vi "motorJoystickcore.vi"(4 "button info":T2, 6 "axis info":T1, 8 "error in":errorcluster[](array[cluster]), 9 "Motor Limits":T3, 10 "Array in":refnum<k7>[](array[refnum])) -> (0 "error out":errorcluster[](array[cluster]), 2 "XYZ position":sgl[](array[numeric]))   [LabVIEW 2014]
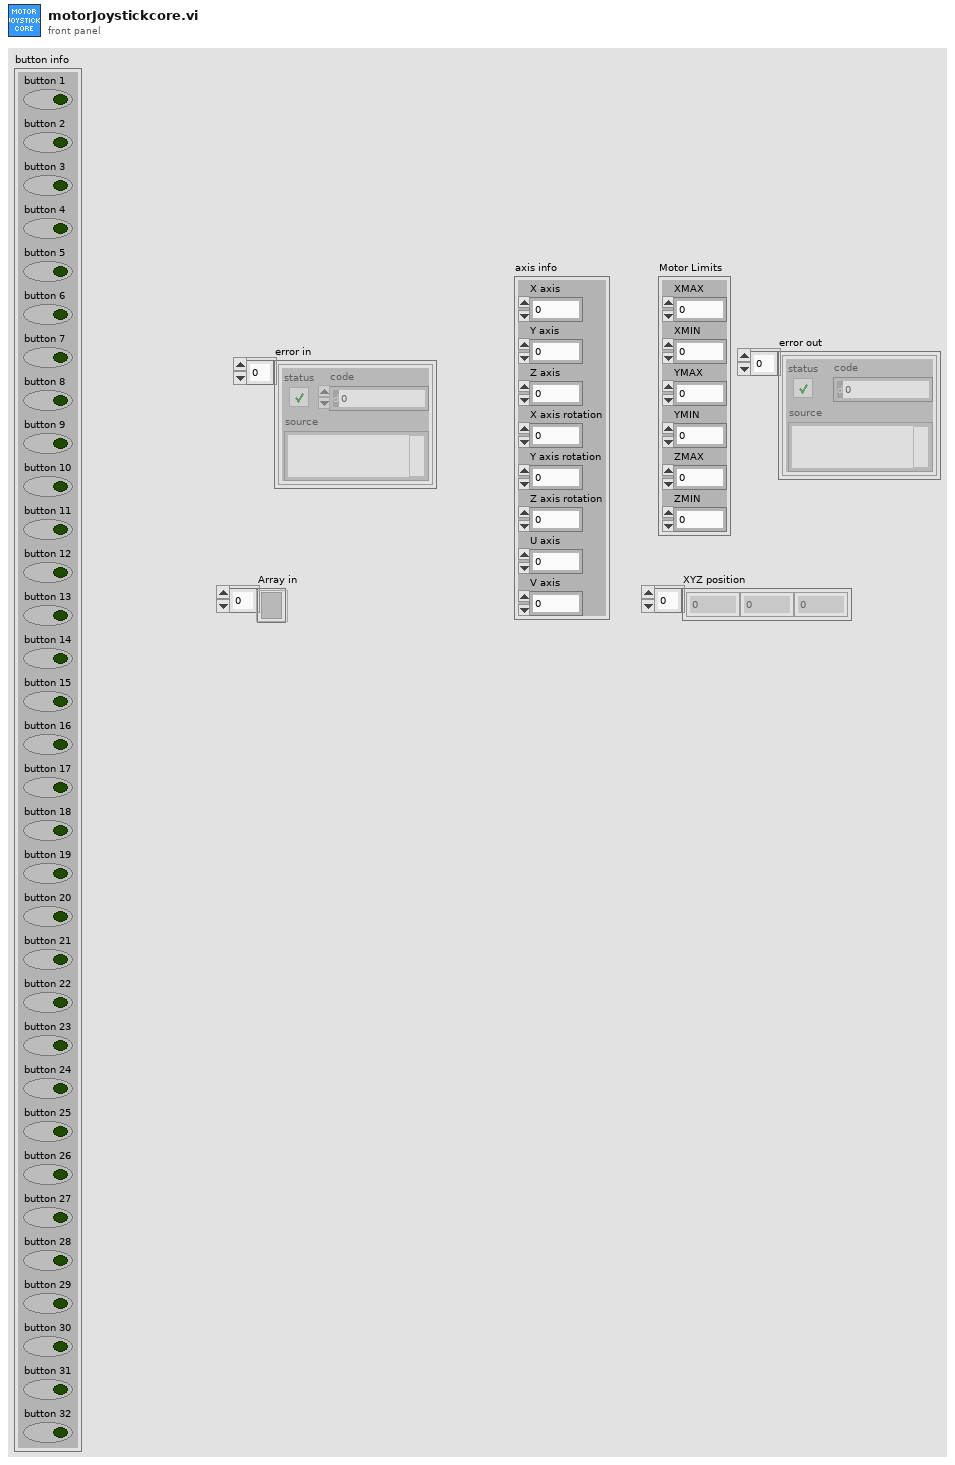
[diagram p1: front panel]
types:
  T1 = cluster{"X axis":i32, "Y axis":i32, "Z axis":i32, "X axis rotation":i32, "Y axis rotation":i32, "Z axis rotation":i32, "U axis":i32, "V axis":i32}
  T2 = cluster{"button 1":bool, "button 2":bool, "button 3":bool, "button 4":bool, "button 5":bool, "button 6":bool, "button 7":bool, "button 8":bool, "button 9":bool, "button 10":bool, "button 11":bool, "button 12":bool, "button 13":bool, "button 14":bool, "button 15":bool, "button 16":bool, "button 17":bool, "button 18":bool, "button 19":bool, "button 20":bool, "button 21":bool, "button 22":bool, "button 23":bool, "button 24":bool, "button 25":bool, "button 26":bool, "button 27":bool, "button 28":bool, "button 29":bool, "button 30":bool, "button 31":bool, "button 32":bool}
  T3 = cluster{"XMAX":sgl, "XMIN":sgl, "YMAX":sgl, "YMIN":sgl, "ZMAX":sgl, "ZMIN":sgl}
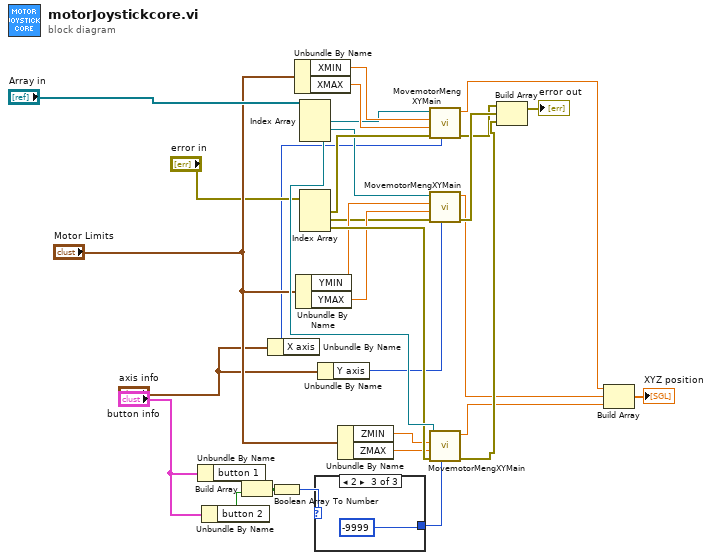
[diagram p0: block diagram]
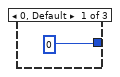
[diagram p2: hidden frame]
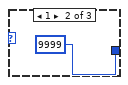
[diagram p3: hidden frame]
diagram:
  n1 = Unbundle By Name("button info") -> ("button 1"=w8:bool)
  n2 = Unbundle By Name("button info") -> ("button 2"=w9:bool)
  n3 = Build Array(w8, w9) -> (w10:bool[])
  n4 = Unbundle By Name("axis info") -> ("X axis"=w6:i32)
  n5 = Boolean Array To Number(Boolean array=w10) -> (number=w11:u32)
  n6 = Unbundle By Name("Motor Limits") -> ("XMIN"=w21:sgl, "XMAX"=w22:sgl)
  n7 = Unbundle By Name("Motor Limits") -> ("YMIN"=w23:sgl, "YMAX"=w24:sgl)
  n8 = Index Array(array="Array in") -> (element #1=w13:refnum<k7>, element #2=w14:refnum<k7>, element #3=w32:refnum<k7>)  [unwired: 3 in]
  n9 = Index Array(array="error in") -> (element #1=w16:errorcluster, element #2=w17:errorcluster, element #3=w29:errorcluster)  [unwired: 3 in]
  n10 = case shown="2" w11 {
    tunnel: [0 ("Y axis") 9999 ("Y axis") -9999 ("Y axis")] -> w12
    frame 0, Default {
    }
    frame 1 {
    }
    frame 2 {
    }
  }
  n11 = Unbundle By Name("axis info") -> ("Y axis"=w7:i32)
  n12 = Unbundle By Name("Motor Limits") -> ("ZMIN"=w25:sgl, "ZMAX"=w26:sgl)
  n13 = call "MovemotorMengXYMain.vi"("Joystick axis"=w6, "error in (no error)"=w16, "XorYMAX"=w22, "XorYMIN"=w21, "Automation Refnum in"=w13) -> ("error out"=w18:errorcluster, "XorYPosition"=w4:sgl)  [unwired: 4 in, 1 out]
  n14 = call "MovemotorMengXYMain.vi"("Joystick axis"=w7, "error in (no error)"=w17, "XorYMAX"=w24, "XorYMIN"=w23, "Automation Refnum in"=w14) -> ("error out"=w19:errorcluster, "XorYPosition"=w3:sgl)  [unwired: 4 in, 1 out]
  n15 = call "MovemotorMengXYMain.vi"("Joystick axis"=w12, "error in (no error)"=w29, "XorYMAX"=w26, "XorYMIN"=w25, "Automation Refnum in"=w32) -> ("error out"=w30:errorcluster, "XorYPosition"=w2:sgl)  [unwired: 4 in, 1 out]
  n16 = Build Array(w18, w19, w30) -> (→"error out":errorcluster[])
  n17 = Build Array(w4, w3, w2) -> (→"XYZ position":sgl[])
